vi "VerifyDeviceIsPresent.vi"(8 "Error In":errorcluster, 11 "Serial Number in":string) -> (0 "Error Out":errorcluster, 3 "Present?":bool)   [LabVIEW 2018, in "Thorlabs.lvlib" / "Thorlabs.lvclass"]
doc: "This VI is used to determine whether the specific Axis Controller with the specified Serial Number is present on the machine.\n\nCreator: Slade Jeppesen\nCreated: 09/29/20"
uses:
  Thorlabs.lvclass
  C:/AME Test Engineering/LabVIEW/PPLs/Axis/DLLs/Thorlabs.MotionControl.DeviceManagerCLI.dll
  PPLs/Axis/DLLs/Thorlabs.MotionControl.DeviceManagerCLI.dll
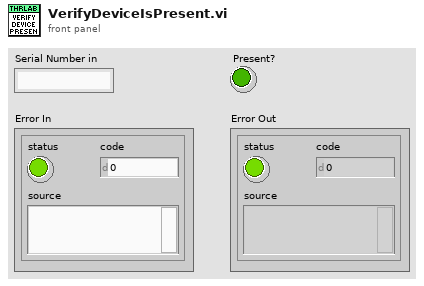
[diagram p1: front panel]
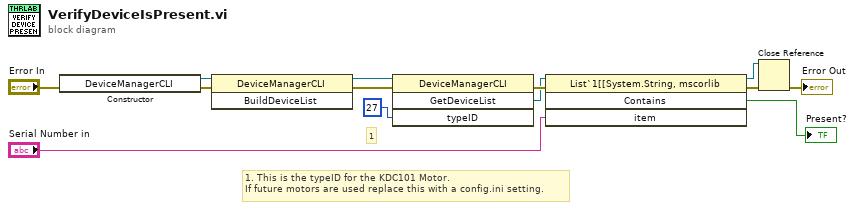
[diagram p0: block diagram]
diagram:
  # "1. This is the typeID for the KDC101 Motor.\nIf future motors are used replace this with a config.ini setting."
  # "1"
  n1 = constructor class="DeviceManagerCLI"(error in="Error In") -> (reference out=w3:refnum<k24>, error out=w1:errorcluster)  [unwired: 2 in, 1 out]
  n2 = invoke class="DeviceManagerCLI" method="BuildDeviceList"(reference=w3, error in=w1) -> (reference out=w12:refnum<k24>, error out=w5:errorcluster)  [unwired: 1 in, 1 out]
  n3 = invoke class="DeviceManagerCLI" method="GetDeviceList"(reference=w12, error in=w5, "typeID"=27) -> (error out=w8:errorcluster, "GetDeviceList"=w7:refnum<k24>)  [unwired: 1 in, 2 out]
  n4 = invoke class="List`1[[System.String, mscorlib" method="Contains"(reference=w7, error in=w8, "item"="Serial Number in") -> (reference out=w10:refnum<k24>, error out=w9:errorcluster, "Contains"=→"Present?":bool)  [unwired: 1 in, 1 out]
  n5 = Close Reference(reference=w10, error in (no error)=w9) -> (error out=→"Error Out":errorcluster)
